vi "Set Server Internal UEs.vi"(10 "Server Internal UEs":T1, 11 "OOP Server in":refnum<class "NW and PSD_server.lvclass">) -> (3 "OOP Server out":refnum<class "NW and PSD_server.lvclass">)   [LabVIEW 2019, in "NW and PSD_server.lvlib" / "NW and PSD_server.lvclass"]
uses:
  NW and PSD_server.lvclass
  typeDefs/Server Internal UEs.ctl
  typeDefs/Server Internal Message.ctl
  NW and PSD_server.lvclass/NW and PSD_server.ctl
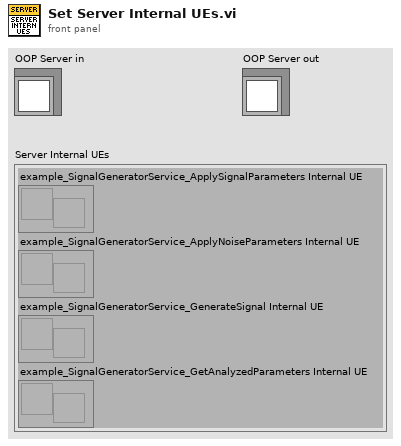
[diagram p1: front panel]
types:
  T1 = typedef "NW and PSD_server.lvlib/NW and PSD_server.lvclass/Server Internal UEs.ctl" = cluster{"example_SignalGeneratorService_ApplySignalParameters Internal UE":refnum<user-event>, "example_SignalGeneratorService_ApplyNoiseParameters Internal UE":refnum<user-event>, "example_SignalGeneratorService_GenerateSignal Internal UE":refnum<user-event>, "example_SignalGeneratorService_GetAnalyzedParameters Internal UE":refnum<user-event>}
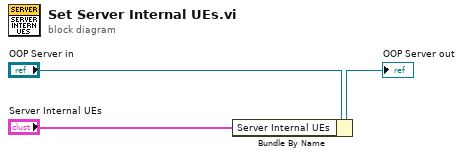
[diagram p0: block diagram]
diagram:
  n1 = Bundle By Name(cluster="OOP Server in", "Server Internal UEs"="Server Internal UEs") -> (→"OOP Server out":refnum<class "NW and PSD_server.lvclass">)
